vi "Save Changes (System).vi"(6 "Remote Timeout (300,000 ms)":u32=300000, 8 "error in (no error)":errorcluster, 11 "Session in":refnum<k21>) -> (0 "error out":errorcluster, 1 "Changes Require Restart":bool, 2 "Detailed Result":string, 3 "Session out":refnum<k21>)   [LabVIEW 2012, in "nisyscfg.lvlib"]
doc: "Writes and saves property changes on a system. Save Changes (System) VI wires into the System Property node where property changes are selected."
uses:
  <vilib>/nisyscfg/nisyscfg.lvlib
  <vilib>/Utility/error.llb/Error Cluster From Error Code.vi
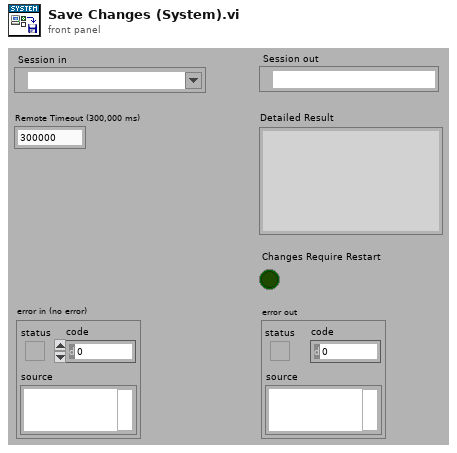
[diagram p1: front panel]
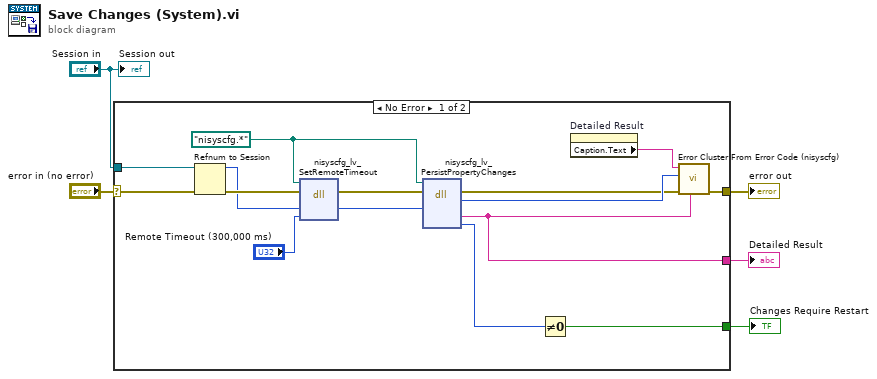
[diagram p0: block diagram]
diagram:
  n1 = case shown="No Error" "error in (no error)" {
    selector: "error in (no error)" -> [w9 w21]
    tunnel: [w18 w21] -> w5
    tunnel: [w10 _] -> w3
    tunnel: "Session in" -> [w7 _]
    tunnel: [w12 _] -> w1
    frame No Error {
      w14 = path "nisyscfg.*" ("path in")
      n2 = Refnum to Session(4:w9, 7:w7) -> (0:w8:errorcluster, 3:w6:u64)
      n3 = dll-call lib="nisyscfg.*" fn="nisyscfg_lv_SetRemoteTimeout" label="SetRemoteTimeout"(path in=w14, error in=w8, "item"=w6, "connectTimeout"="Remote Timeout (300,000 ms)") -> (error out=w17:errorcluster, "item"=w15:u64)  [unwired: 1 in, 3 out]
      n4 = dll-call lib="nisyscfg.*" fn="nisyscfg_lv_PersistPropertyChanges" label="nisysPersistPropertyChangesLV"(path in=w14, error in=w17, "item"=w15) -> (error out=w19:errorcluster, "status"=w20:i32, "detailed result"=w10:string, "requiresRestart"=w13:u8)  [unwired: 1 in, 4 out]
      n5 = Not Equal To 0?(x=w13) -> (x != 0?=w12:bool)
      n6 = property on="Detailed Result" class="Str"() -> ("Caption.Text"=w11:string)  [unwired: 2 in, 2 out]
      n7 = call <vilib>:"Error Cluster From Error Code (nisyscfg).vi"("Details String"=w10, "error in (no error)"=w19, "Error Code (0)"=w20, "Details Caption"=w11) -> ("error out"=w18:errorcluster)  [unwired: 7 in]
    }
    frame Error {
    }
  }
  "error out" <- w5
  "Detailed Result" <- w3
  "Changes Require Restart" <- w1
  "Session out" <- "Session in"
